vi "Parse GSV.vi"(8 "error in (no error)":errorcluster, 10 "Message":refnum<class "NMEA Message.lvclass">, 11 "nmea in":refnum<class "nmea.lvclass">) -> (0 "error out":errorcluster, 3 "nmea out":refnum<class "nmea.lvclass">)   [LabVIEW 2020, in "nmea.lvlib" / "nmea.lvclass"]
uses:
  nmea.lvclass
  message/NMEA Message.lvclass
  nmea.lvclass/nmea.ctl
  Satellite.ctl
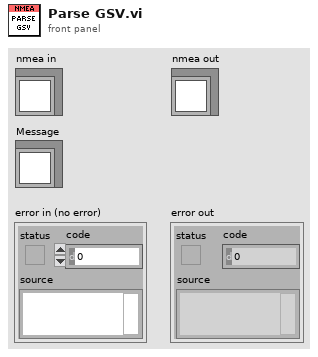
[diagram p1: front panel]
types:
  T1 = typedef "nmea.lvlib/nmea.lvclass/Ref Data.ctl" = cluster{"Latitude":dbl, "Longitude":dbl, "Time":T2, "Status":string, "Speed":dbl, "Course":dbl, "Mag Var":dbl, "Var Dir":string, "Mode":string, "Satellites":T3[], "Next Satellites":T3[], "Active PRNs":i32[], "Fix Type":T4, "DOP":T5, "Fix Mode":T6, "Altitude":dbl, "Geoid":dbl}
  T2 = typedef "LVDateTimeRec.ctl" = cluster{"fractional second":dbl, "second":i32, "minute":i32, "hour":i32, "day of month":i32, "month":i32, "year":i32, "day of week":i32, "day of year":i32, "DST":i32}
  T3 = typedef "nmea.lvlib/nmea.lvclass/Satellite.ctl" = cluster{"PRN":u8, "Channel":u8, "Elevation":u8, "Azimuth":u16, "SNR":u8, "Active":bool}
  T4 = typedef "nmea.lvlib/nmea.lvclass/Fix Type.ctl" = enum16{"N/A", "None", "2D", "3D"}
  T5 = typedef "nmea.lvlib/nmea.lvclass/DOP.ctl" = cluster{"P":dbl, "H":dbl, "V":dbl}
  T6 = typedef "nmea.lvlib/nmea.lvclass/Fix Mode.ctl" = enum16{"Manual", "Auto 2/3D"}
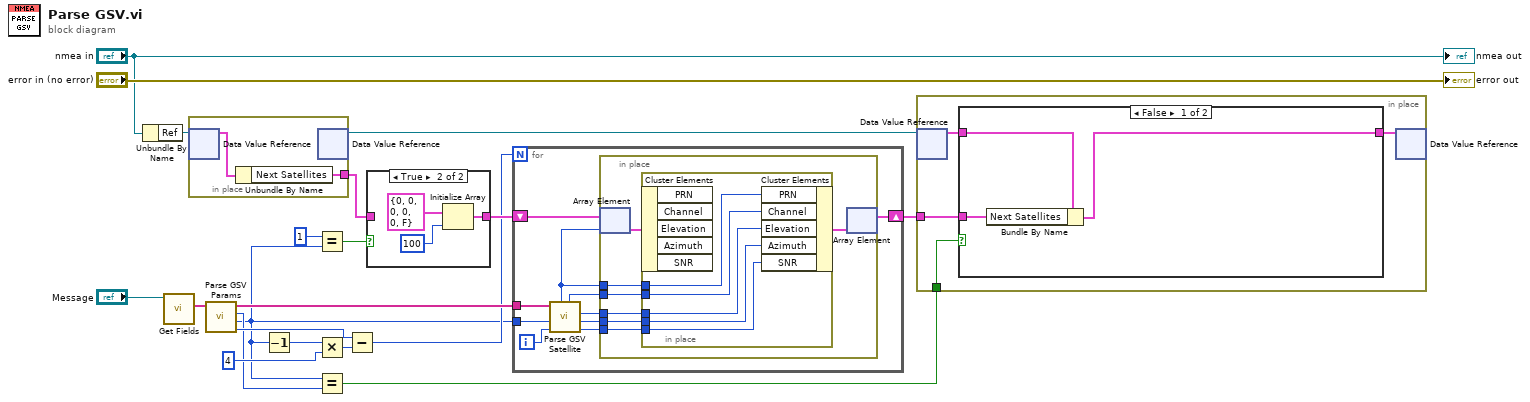
[diagram p0: block diagram]
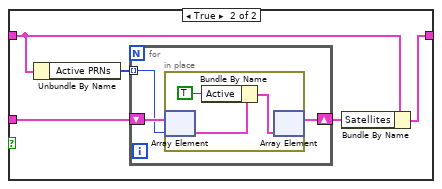
[diagram p2: hidden frame]
diagram:
  n1 = Unbundle By Name("nmea in") -> ("Ref"=w16:refnum<data-value>)
  n2 = call "Get Fields.vi"("NMEA Message in"="Message") -> ("Fields"=w18:string[])  [unwired: 8 in, 2 out]
  n3 = in-place {
    in-place-border: [w21] -> w13
    n4 = in-place-dvr #1(w16) -> (w22:T1)  [unwired: 1 out]
    n5 = Unbundle By Name(w22) -> ("Next Satellites"=w21:T3[])
    n6 = in-place-dvr #1() -> (w4:refnum<data-value>)  [unwired: 1 in, 1 out]
  }
  n7 = call "Parse GSV Params.vi"("Fields In"=w18) -> ("Total SVs"=w9:i32, "Message Num"=w5:i32, "Total Messages"=w7:i32, "Fields"=w8:string[])  [unwired: 7 in]
  n8 = Decrement(x=w5) -> (x-1=w1:i32)
  n9 = Equal?(x=1, y=w5) -> (x = y?=w12:bool)
  n10 = Multiply(x=w1, y=4) -> (x*y=w10:i32)
  n11 = Equal?(x=w5, y=w7) -> (x = y?=w2:bool)
  n12 = Subtract(x=w9, y=w10) -> (x-y=w6:i32)
  n13 = case shown="True" w12 {
    tunnel: w13 -> [w23 _]
    tunnel: [w23 w24] -> w11
    frame False {
    }
    frame True {
      n14 = Initialize Array(T3 {"PRN"=0, "Channel"=0, "Elevation"=0, "Azimuth"=0, "SNR"=0, "Active"=FALSE} ("Satellite"), 100 ("dimension size")) -> (w24:T3[])
    }
  }
  n15 = for {
    N: w6 -> [_]
    shift-right: [w28] -> w3
    shift-left: w11 -> [w36]
    tunnel: w8 -> [w35]
    tunnel: w5 -> [w34]
    i -> [w33]
    n16 = call "Parse GSV Satellite.vi"("Message SV Num"=w33, "Message Num"=w34, "Fields In"=w35) -> ("SNR"=w29:i32, "Azimuth"=w30:i32, "Elevation"=w31:i32, "Channel"=w32:i32, "PRN"=w27:i32)  [unwired: 3 in, 1 out]
    n17 = in-place {
      in-place-border: w32 -> [w42]
      in-place-border: w31 -> [w41]
      in-place-border: w30 -> [w40]
      in-place-border: w29 -> [w39]
      in-place-border: w27 -> [w37]
      n18 = in-place-array #2(w36, w27) -> (w43:T3)
      n19 = in-place {
        in-place-border: w42 -> [w48]
        in-place-border: w41 -> [w47]
        in-place-border: w40 -> [w46]
        in-place-border: w39 -> [w45]
        in-place-border: w37 -> [w44]
        n20 = in-place-cluster #3(w43) -> ()  [unwired: 5 out]
        n21 = in-place-cluster #3("PRN"=w44, "Channel"=w48, "Elevation"=w47, "Azimuth"=w46, "SNR"=w45) -> (w38:T3)
      }
      n22 = in-place-array #2(w38) -> (w28:T3[])  [unwired: 1 out]
    }
  }
  n23 = in-place {
    in-place-border: w3 -> [w52]
    in-place-border: w2 -> [w49]
    n24 = in-place-dvr #4(w4) -> (w51:T1)  [unwired: 1 out]
    n25 = case shown="False" w49 {
      tunnel: w52 -> [w54 w58]
      tunnel: w51 -> [w55 w59]
      tunnel: [w53 w60] -> w50
      frame False {
        n26 = Bundle By Name(cluster=w55, "Next Satellites"=w54) -> (w53:T1)
      }
      frame True {
        n27 = Unbundle By Name(w59) -> ("Active PRNs"=w57:i32[])
        n28 = for {
          tunnel: w57 -> [w62] mode=indexing
          shift-right: [w61] -> w56
          shift-left: w58 -> [w63]
          n29 = in-place {
            n30 = in-place-array #5(w63, w62) -> (w66:T3)
            n31 = Bundle By Name(cluster=w66, "Active"=TRUE) -> (w64:T3)
            n32 = in-place-array #5(w64) -> (w61:T3[])  [unwired: 1 out]
          }
        }
        n33 = Bundle By Name(cluster=w59, "Satellites"=w56) -> (w60:T1)
      }
    }
    n34 = in-place-dvr #4(w50) -> ()  [unwired: 2 out]
  }
  "error out" <- "error in (no error)"
  "nmea out" <- "nmea in"
